vi "Save Plugin Scripts.vi"(8 "error in (no error)":errorcluster, 11 "TreeControl in":refnum<vi>) -> (0 "error out":errorcluster, 1 "New Tags After Save":string[](array[string]), 3 "TreeControl out":refnum<vi>)   [LabVIEW 2018]
uses:
  <vilib>/Utility/config.llb/NI_LVConfig.lvlib
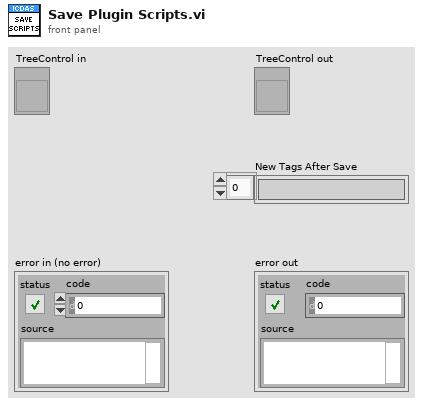
[diagram p1: front panel]
types:
  T1 = typedef "Plugin Tree Tag.ctl" = cluster{"ItemType":T2, "Name":string, "Path":path, "Script":string[]}
  T2 = typedef "Plugins Tree Item Type.ctl" = enum16{"Plugin", "Instrument", "INI File", "INI Script"}
  T3 = typedef "NI_LVConfig.lvlib/Config Data RefNum.ctl" = refnum<k1>
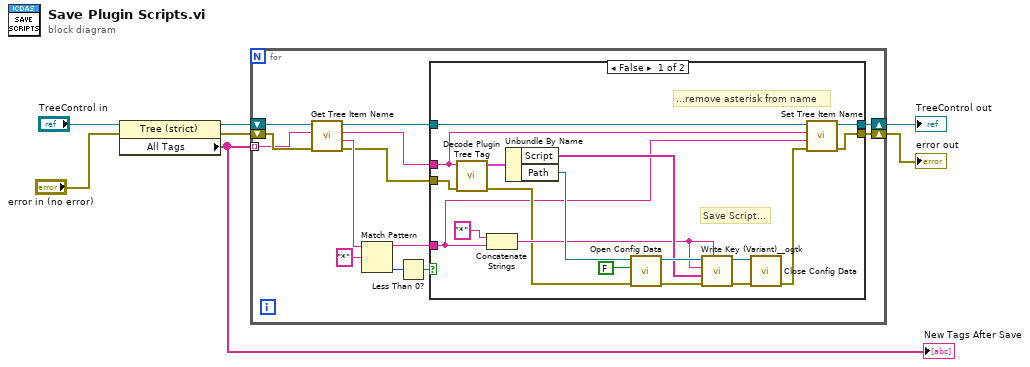
[diagram p0: block diagram]
diagram:
  n1 = property class="Tree (strict)"(reference="TreeControl in", error in="error in (no error)") -> (reference out=w4:refnum<vi>, error out=w5:errorcluster, "All Tags"=w3:string[])
  "New Tags After Save" <- w3
  n2 = for {
    tunnel: w3 -> [w18] mode=indexing
    shift-right: [w10] -> w7
    shift-left: w5 -> [w19]
    shift-right: [w8] -> w1
    shift-left: w4 -> [w20]
    n3 = call "Get Tree Item Name.vi"("error in (no error)"=w19, "Tag"=w18, "TreeControl in"=w20) -> ("error out"=w12:errorcluster, "Item Name"=w17:string, "Tag out"=w13:string, "TreeControl out"=w9:refnum<vi>)  [unwired: 5 in]
    n4 = Match Pattern(string=w17, regular expression="*") -> (before substring=w11:string, offset past match=w15:i32)  [unwired: 1 in, 2 out]
    n5 = Less Than 0?(x=w15) -> (x < 0?=w14:bool)
    n6 = case shown="False" w14 {
      tunnel: w13 -> [w23 _]
      tunnel: w12 -> [w38 w40]
      tunnel: w11 -> [w24 _]
      tunnel: [w21 w40] -> w10
      tunnel: w9 -> [w26 w39]
      tunnel: [w25 w39] -> w8
      frame False {
        # "Save Script..."
        # "...remove asterisk from name"
        n7 = call "Decode Plugin Tree Tag.vi"("error in (no error)"=w38, "Tag"=w23) -> ("error out"=w27:errorcluster, "Plugin Tree Tag"=w32:T1)  [unwired: 8 in]
        n8 = Concatenate Strings("*" ("string"), w24) -> (w28:string)
        n9 = Unbundle By Name(w32) -> ("Script"=w31:string[], "Path"=w29:path)
        n10 = call <vilib>:"Open Config Data.vi"("error in (no error)"=w27, "create file if necessary (T)"=FALSE, "configuration file path"=w29) -> ("error out"=w36:errorcluster, "refnum"=w34:T3)  [unwired: 6 in, 1 out]
        n11 = call <userlib>:"Write Key (Variant)__ogtk.vi"("section"=w28, "error in (no error)"=w36, "key-value"=w31, "key (optional)"=w28, "refnum"=w34) -> ("error out"=w35:errorcluster, "refnum out"=w33:T3)  [unwired: 5 in]
        n12 = call <vilib>:"Close Config Data.vi"("error in (no error)"=w35, "refnum"=w33) -> ("error out"=w22:errorcluster)  [unwired: 8 in, 1 out]
        n13 = call "Set Tree Item Name.vi"("error in (no error)"=w22, "Item Name"=w24, "Tag"=w23, "TreeControl in"=w26) -> ("error out"=w21:errorcluster, "TreeControl out"=w25:refnum<vi>)  [unwired: 5 in, 1 out]
      }
      frame True {
      }
    }
  }
  "error out" <- w7
  "TreeControl out" <- w1
